vi "filenameToDOS.vi"(8 "error in (no error)":errorcluster, 11 "file name":string) -> (0 "error out":errorcluster, 3 "8.3 filename":string)   [LabVIEW 2013]
panel:
  # "works just by shortening; does not add ~ or anything helpful like that"
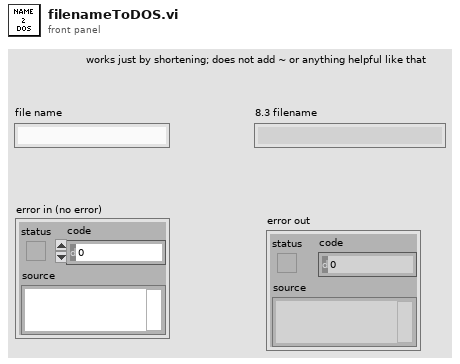
[diagram p1: front panel]
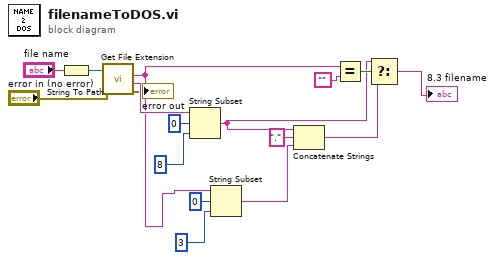
[diagram p0: block diagram]
diagram:
  n1 = String To Path(string="file name") -> (path=w16:path)
  n2 = call <vilib>:"Get File Extension.vi"("error in (no error)"="error in (no error)", "file"=w16) -> ("error out"=→"error out":errorcluster, "filename without extension"=w14:string, "lowercase file extension"=w6:string)  [unwired: 6 in, 1 out]
  n3 = String Subset(string=w14, offset (0)=0, length (rest)=8 ("length (rest)")) -> (substring=w4:string)
  n4 = String Subset(string=w6, offset (0)=0, length (rest)=3 ("length (rest)")) -> (substring=w9:string)
  n5 = Concatenate Strings(w4, "." ("string"), w9) -> (w3:string)
  n6 = Equal?(x=w6, y="") -> (x = y?=w5:bool)
  n7 = Select(t=w4, s=w5, f=w3) -> (s? t:f=→"8.3 filename":string)
